vi "Test PCAN-USB Read Raw Frame EXCEL.vi"(11 "Test Case In":refnum<class "Test Communicator.lvclass">) -> (0 "error out":errorcluster, 3 "Test Case Out":refnum<class "Test Communicator.lvclass">)   [LabVIEW 2024, in "Test Communicator.lvclass"]
uses:
  Test Communicator.lvclass
  Test Communicator.lvclass/Test Communicator.ctl
  <vilib>/Astemes/LUnit/Test Case.lvclass
  Source/Communicator/Communicator.lvclass
  Source/Interfaces/IMessage/IMessage.lvclass
  Source/Configure Strategies/PCAN-USB Strategies/PCAN-USB Read-Write Raw CAN Frame Strategy/PCAN Read-Write Raw CAN Frame Strategy.lvclass
  Source/Configure Strategies/PCAN-USB Strategies/PCAN-USB Base Strategy/PCAN Base Strategy.lvclass
  D:/git/HAL/Source/Interfaces/IConfigure/IConfigure.lvclass
  D:/git/HAL/Source/Interfaces/IClose/IClose.lvclass
  D:/git/HAL/Source/Interfaces/IInitialize/IInitialize.lvclass
  D:/git/HAL/HAL-Devices/Source/Configure Strategies/PCAN-USB Strategies/PCAN-USB Base Strategy/PCAN Base Strategy.lvclass
  D:/git/HAL/Source/Interfaces/ICommunicate/ICommunicate.lvclass
  D:/git/HAL/Source/Interfaces/IRunnable/IRunnable.lvclass
  D:/git/HAL/Source/Interfaces/IValidate Configuration/IValidate Configuration.lvclass
panel:
  out "Timestamp":timestamp
  out "Data":u8[](array[numeric]) format="%.0x"
  out "Identifier":string
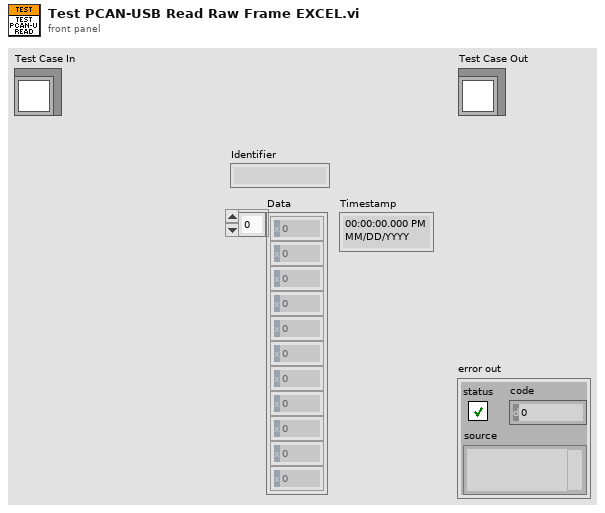
[diagram p1: front panel]
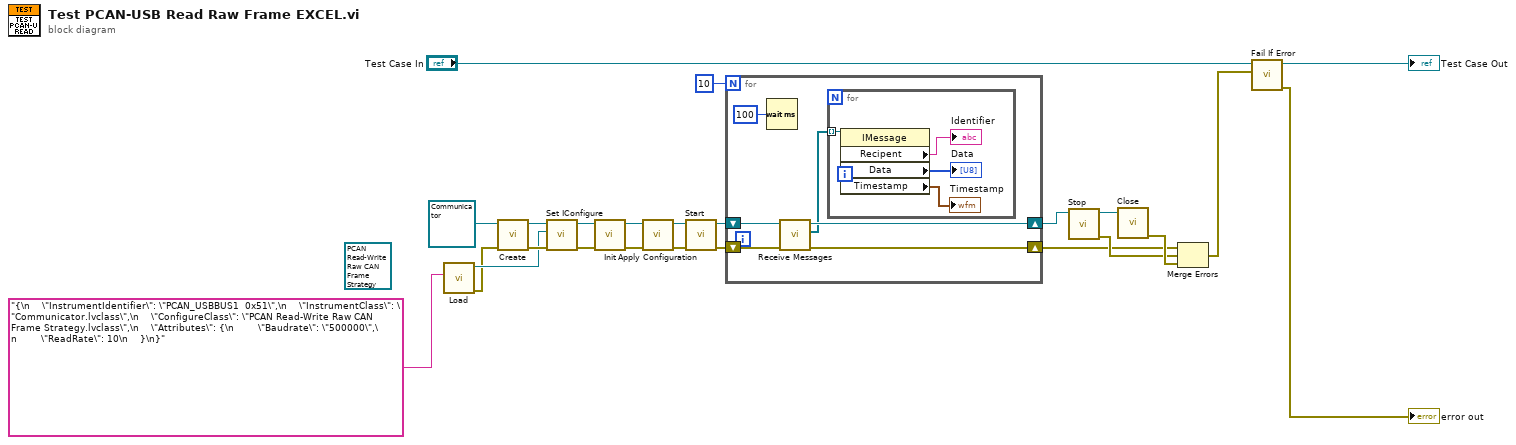
[diagram p0: block diagram]
diagram:
  (unwired) refnum<class "PCAN Read-Write Raw CAN Frame Strategy.lvclass"> refnum ("PCAN-USB Read-Write Raw CAN Frame Strategy")
  n1 = call-dynamic "Load.vi"("Source"="{\n    \"InstrumentIdentifier\": \"PCAN_USBBUS1  0x51\",\n    \"InstrumentClass\": \"Communicator.lvclass\",\n    \"ConfigureClass\": \"PCAN Read-Write Raw CAN Frame Strategy.lvclass\",\n    \"Attributes\": {\n        \"Baudrate\": \"500000\",\n        \"ReadRate\": 10\n    }\n}") -> ("error out"=w3:errorcluster, "PCAN-USB Read-Write Raw CAN Frame Strategy out"=w20:refnum<class "PCAN Base Strategy.lvclass">)  [unwired: 9 in]
  n2 = call-dynamic "Create.vi"("Error In"=w3, "reference in"=refnum<class "Communicator.lvclass"> refnum ("NI9862 in")) -> ("Error Out"=w21:errorcluster, "reference out"=w11:refnum<class "Communicator.lvclass">)  [unwired: 8 in]
  n3 = call-dynamic "Set IConfigure.vi"("Error In"=w21, "IConfigure"=w20, "Communicator in"=w11) -> ("Error Out"=w19:errorcluster, "Communicator out"=w18:refnum<class "Communicator.lvclass">)  [unwired: 7 in]
  n4 = call-dynamic "Init.vi"("Error In"=w19, "Communicator in"=w18) -> ("Error Out"=w17:errorcluster, "Communicator out"=w16:refnum<class "Communicator.lvclass">)  [unwired: 8 in]
  n5 = call-dynamic "Apply Configuration.vi"("Error In"=w17, "Communicator in"=w16) -> ("Error Out"=w8:errorcluster, "Communicator out"=w9:refnum<class "Communicator.lvclass">)  [unwired: 8 in]
  n6 = call-dynamic "Start.vi"("Error In"=w8, "Communicator in"=w9) -> ("Error Out"=w13:errorcluster, "Communicator out"=w14:refnum<class "Communicator.lvclass">)  [unwired: 8 in]
  n7 = for {
    N: 10 -> [_]
    shift-right: [w28] -> w12
    shift-left: w14 -> [w30]
    shift-right: [w27] -> w4
    shift-left: w13 -> [w29]
    n8 = Wait (ms)(milliseconds to wait=u32 100) -> ()  [unwired: 1 out]
    n9 = call-dynamic "Receive Messages.vi"("Error In"=w29, "Communicator in"=w30) -> ("Error Out"=w27:errorcluster, "Messages"=w26:refnum<class "IMessage.lvclass">[], "Communicator out"=w28:refnum<class "Communicator.lvclass">)  [unwired: 7 in]
    n10 = for {
      tunnel: w26 -> [w34] mode=indexing
      n11 = property class="IMessage"(reference=w34) -> ("Recipent"=→"Identifier":string, "Data"=→"Data":u8[], "Timestamp"=→"Timestamp":timestamp)  [unwired: 1 in, 2 out]
    }
  }
  n12 = call-dynamic "Stop.vi"("Communicator in"=w12) -> ("Error Out"=w5:errorcluster, "Communicator out"=w10:refnum<class "Communicator.lvclass">)  [unwired: 9 in]
  n13 = call-dynamic "Close.vi"("Communicator in"=w10) -> ("Error Out"=w7:errorcluster)  [unwired: 9 in, 1 out]
  n14 = Merge Errors(w4, w5, w7) -> (w6:errorcluster)
  n15 = call <vilib>:"Fail If Error.vi"("Assert error"=w6, "LUnit Test Case In"="Test Case In") -> ("error out"=→"error out":errorcluster, "LUnit Test Case Out"=→"Test Case Out":refnum<class "Test Communicator.lvclass">)  [unwired: 8 in]
